vi "remove pre post build from project.vi"(8 "error in (no error)":errorcluster, 11 "pre and post build refs":refnum<vi>[](array[refnum])) -> (0 "error out":errorcluster)   [LabVIEW 2024]
doc: "If the reference is valid, removes the pre and post build action vis from project"
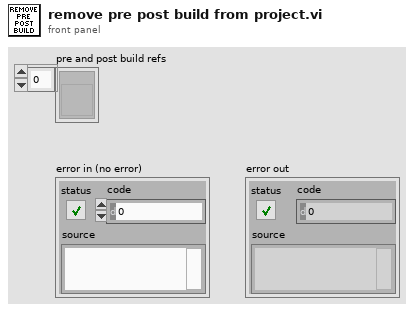
[diagram p1: front panel]
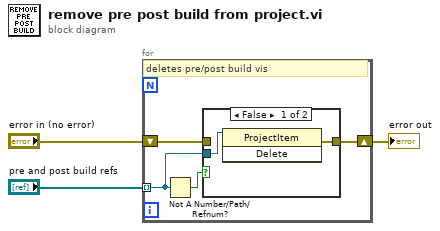
[diagram p0: block diagram]
diagram:
  n1 = for {
    tunnel: "pre and post build refs" -> [w5] mode=indexing
    shift-right: [w6] -> w2
    shift-left: "error in (no error)" -> [w7]
    # "deletes pre/post build vis"
    n2 = Not A Number/Path/Refnum?(number/path/refnum=w5) -> (NaN/Path/Refnum?=w4:bool)
    n3 = case shown="False" w4 {
      tunnel: w7 -> [_ w10]
      tunnel: w5 -> [w9 _]
      tunnel: [w8 w10] -> w6
      frame False {
        n4 = invoke class="ProjectItem" method="Delete"(reference=w9) -> (error out=w8:errorcluster)  [unwired: 2 in, 2 out]
      }
      frame True {
      }
    }
  }
  "error out" <- w2
